vi "Update Busy.vi"(7 "Assert After (500 ms)":u32=500, 8 "error in (no error)":errorcluster, 10 "Busy (False)":bool, 11 "BUSY Ref":refnum<vi>) -> (0 "error out":errorcluster)   [LabVIEW 2025, in "I2C Bus Monitor UI.lvlib"]
uses:
  I2C Bus Monitor UI.lvlib
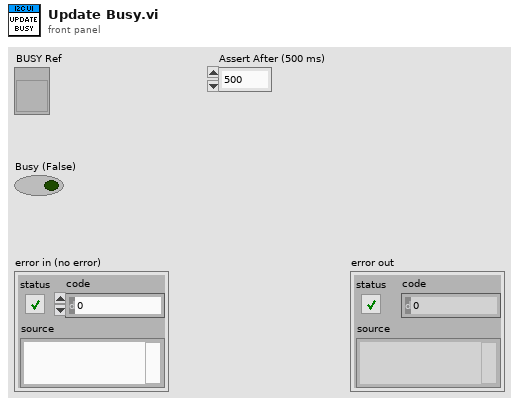
[diagram p1: front panel]
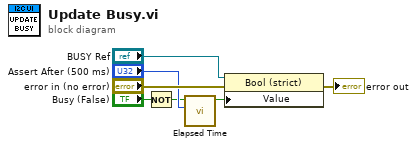
[diagram p0: block diagram]
diagram:
  n1 = Not(x="Busy (False)") -> (.not. x?=w1:bool)
  n2 = call "Elapsed Time.vi"("Target (ms)"="Assert After (500 ms)", "Reset"=w1) -> ("Elapsed"=w5:bool)  [unwired: 8 in, 1 out]
  n3 = property class="Bool (strict)"(reference="BUSY Ref", error in="error in (no error)", "Value"=w5) -> (error out=→"error out":errorcluster)  [unwired: 1 out]
